vi "Read Center Orientation.vi"(7 "Part Type":T1, 8 "error in":errorcluster, 9 "slot":i32, 10 "chuck":i32, 11 "Config Manager in":refnum<class "Config Manager Class.lvclass">) -> (0 "error out":errorcluster, 2 "Location/Orientation":T2, 3 "Config Manager out":refnum<class "Config Manager Class.lvclass">)   [LabVIEW 2011, in "Config Manager Class.lvclass"]
uses:
  Config Manager Class.lvclass
  Utils/Type Definitions/Position_Orientation.ctl
  Vec3d Class/Vec3d Class.lvclass
  Orient3d Class/Orient3d Class.lvclass
  Type Definitions/Part Type.ctl
  Config Manager Class.lvclass/Config Manager Class.ctl
  <vilib>/Utility/config.llb/Read Key (String).vi
  <vilib>/Utility/config.llb/NI_LVConfig.lvlib
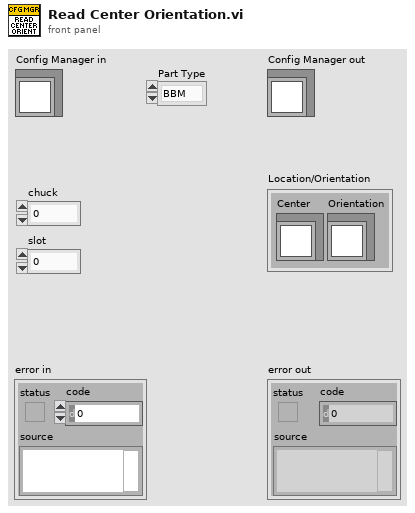
[diagram p1: front panel]
types:
  T1 = typedef "Part Type.ctl" = enum16{"BBM", "HDI", "BARE HDI", "GLUERESERVOIR", "STAMP_1", "STAMP_2", "STAMP_3", "STAMP_4", "STAMP_5", "WEIGHT_1", "WEIGHT_2", "WEIGHT_3", "WEIGHT_4", "WEIGHT_5", "WEIGHT_6", "WEIGHT_7", "WEIGHT_8", "PICKER_TOOL", "GRABER_TOOL"}
  T2 = typedef "Position_Orientation.ctl" = cluster{"Center":refnum<class "Vec3d Class.lvclass">, "Orientation":refnum<class "Orient3d Class.lvclass">}
  T3 = typedef "NI_LVConfig.lvlib/Config Data RefNum.ctl" = refnum<k1>
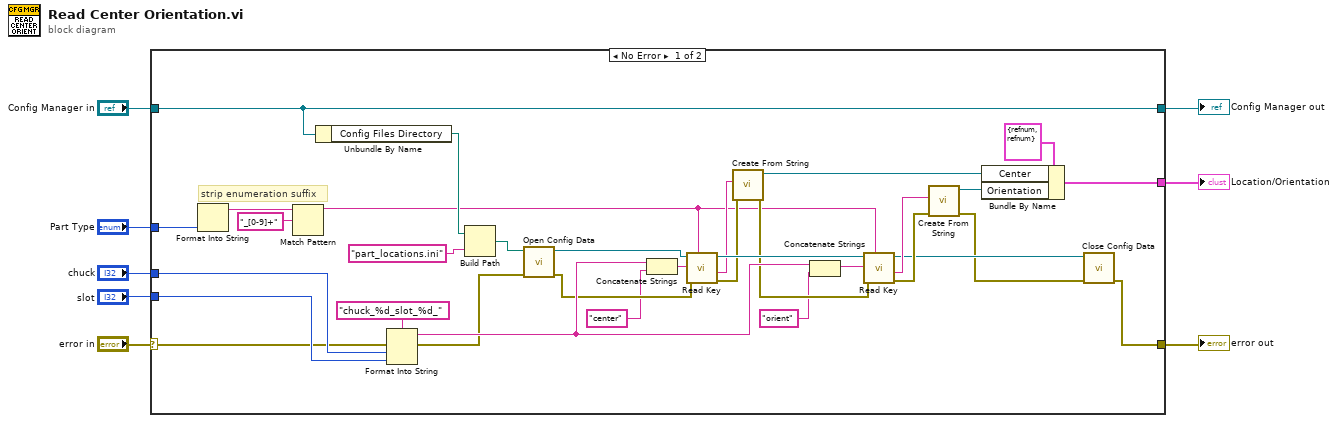
[diagram p0: block diagram]
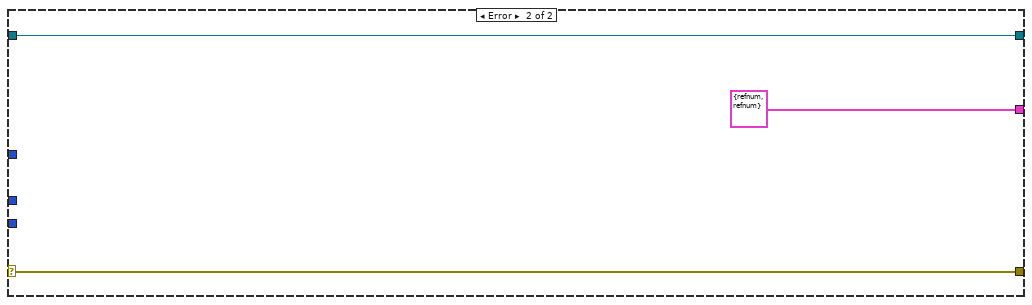
[diagram p2: hidden frame]
diagram:
  n1 = case shown="No Error" "error in" {
    selector: "error in" -> [w15 w44]
    tunnel: [w13 w44] -> w7
    tunnel: [w20 w43] -> w5
    tunnel: "Config Manager in" -> [w20 w43]
    tunnel: "Part Type" -> [w18 _]
    tunnel: "chuck" -> [w17 _]
    tunnel: "slot" -> [w16 _]
    tunnel: [w12 T2 {"Center"=refnum, "Orientation"=refnum} ("Location/Orientation")] -> w1
    frame No Error {
      # "strip enumeration suffix"
      n2 = Format Into String(w18) -> (resulting string=w11:string)  [unwired: 3 in, 1 out]
      n3 = Match Pattern(string=w11, regular expression="_[0-9]+") -> (before substring=w9:string)  [unwired: 1 in, 3 out]
      n4 = Unbundle By Name(w20) -> ("Config Files Directory"=w19:path)
      n5 = Format Into String(format string="chuck_%d_slot_%d_", error in=w15, w17, w16) -> (resulting string=w36:string, error out=w14:errorcluster)  [unwired: 1 in]
      n6 = Build Path(base path=w19, name or relative path="part_locations.ini") -> (appended path=w23:path)
      n7 = call <vilib>:"Open Config Data.vi"("error in (no error)"=w14, "configuration file path"=w23) -> ("error out"=w27:errorcluster, "refnum"=w28:T3)  [unwired: 7 in, 1 out]
      n8 = Concatenate Strings(w36, "center" ("string")) -> (w38:string)
      n9 = call-poly <vilib>:"Read Key.vi"("section"=w9, "error in (no error)"=w27, "key"=w38, "refnum"=w28) -> ("error out"=w33:errorcluster, "value"=w35:string, "refnum out"=w40:T3)  [unwired: 4 in, 1 out]
      n10 = call "Create From String.vi"("error in"=w33, "Input String"=w35) -> ("error out"=w32:errorcluster, "Vec3d out"=w34:refnum<class "Vec3d Class.lvclass">)  [unwired: 8 in]
      n11 = Concatenate Strings(w36, "orient" ("string")) -> (w37:string)
      n12 = call-poly <vilib>:"Read Key.vi"("section"=w9, "error in (no error)"=w32, "key"=w37, "refnum"=w40) -> ("error out"=w30:errorcluster, "value"=w31:string, "refnum out"=w26:T3)  [unwired: 4 in, 1 out]
      n13 = call "Create From String.vi"("error in"=w30, "Input String"=w31) -> ("error out"=w25:errorcluster, "Orient3d out"=w29:refnum<class "Orient3d Class.lvclass">)  [unwired: 8 in]
      n14 = Bundle By Name(cluster=T2 {"Center"=refnum, "Orientation"=refnum} ("Location/Orientation"), "Center"=w34, "Orientation"=w29) -> (w12:T2)
      n15 = call <vilib>:"Close Config Data.vi"("error in (no error)"=w25, "refnum"=w26) -> ("error out"=w13:errorcluster)  [unwired: 8 in, 1 out]
    }
    frame Error {
    }
  }
  "error out" <- w7
  "Config Manager out" <- w5
  "Location/Orientation" <- w1
